vi "StrikerNormal.vi"(6 "atacando ao contrário?":bool=TRUE, 8 "IA Input":T1, 9 "balls":T4[](array[typedef])=[{"x"=-2165.869384765625, "y"=510.4085693359375, "timestamp"=timestamp(2082758857.4639893 s since 1904-01-01), "Vel_x"=0.0, "Vel_y"=0.0}], 10 "Field Size in":T5={"line_width"=10, "field_length"=6000, "field_width"=4000, "boundary_width"=250, "referee_width"=425, "goal_width"=700, "goal_depth"=180, "goal_wall_width"=20, "center_circle_radius"=500, "defense_radius"=500, "defense_stretch"=350, "free_kick_from_defense_dist"=700, "penalty_spot_from_field_line_dist"=450, "penalty_line_from_spot_dist"=350}, 11 "Robot in":T2={"id"=5, "function"=enum."Attacker", "x"=-1842.5054931640625, "y"=520.60986328125, "orientation"=-2.7555055618286133, "v_tangent"=0.0, "v_normal"=0.0, "v_ang"=0.0, "kick_x"=0.0, "kick_z"=0.0, "dribble"=FALSE, "Timestamp"=timestamp(2082758857.4639893 s since 1904-01-01), "dest_x"=0.0, "dest_y"=0.0, "dest_orientation"=0.0, "estimatives"={"est_v_tangent"=0.0, "est_v_normal"=0.0, "est_vx"=0.0, "est_vy"=0.0}}) -> (2 "Robot out":T2={"id"=5, "function"=enum."Attacker", "x"=-1842.5054931640625, "y"=520.60986328125, "orientation"=-2.7555055618286133, "v_tangent"=-0.08361641967936218, "v_normal"=-0.20513016702014014, "v_ang"=0.24456003022714357, "kick_x"=0.0, "kick_z"=0.0, "dribble"=FALSE, "Timestamp"=timestamp(2082758857.4639893 s since 1904-01-01), "dest_x"=0.0, "dest_y"=0.0, "dest_orientation"=0.0, "estimatives"={"est_v_tangent"=0.0, "est_v_normal"=0.0, "est_vx"=0.0, "est_vy"=0.0}})   [LabVIEW 2016]
uses:
  Core/AI Robot.ctl
  Functions Enum.ctl
  Core/Field Size.ctl
  Core/AI Ball.ctl
  Core/AI Input.ctl
  Core/AI Judge.ctl
  Command Enum.ctl
panel:
  in  "dist 2":dbl=700.0
  out "sentido":dbl
  in  "dist":dbl=700.0
  out "Yattacker":dbl
  out "Xattacker":dbl
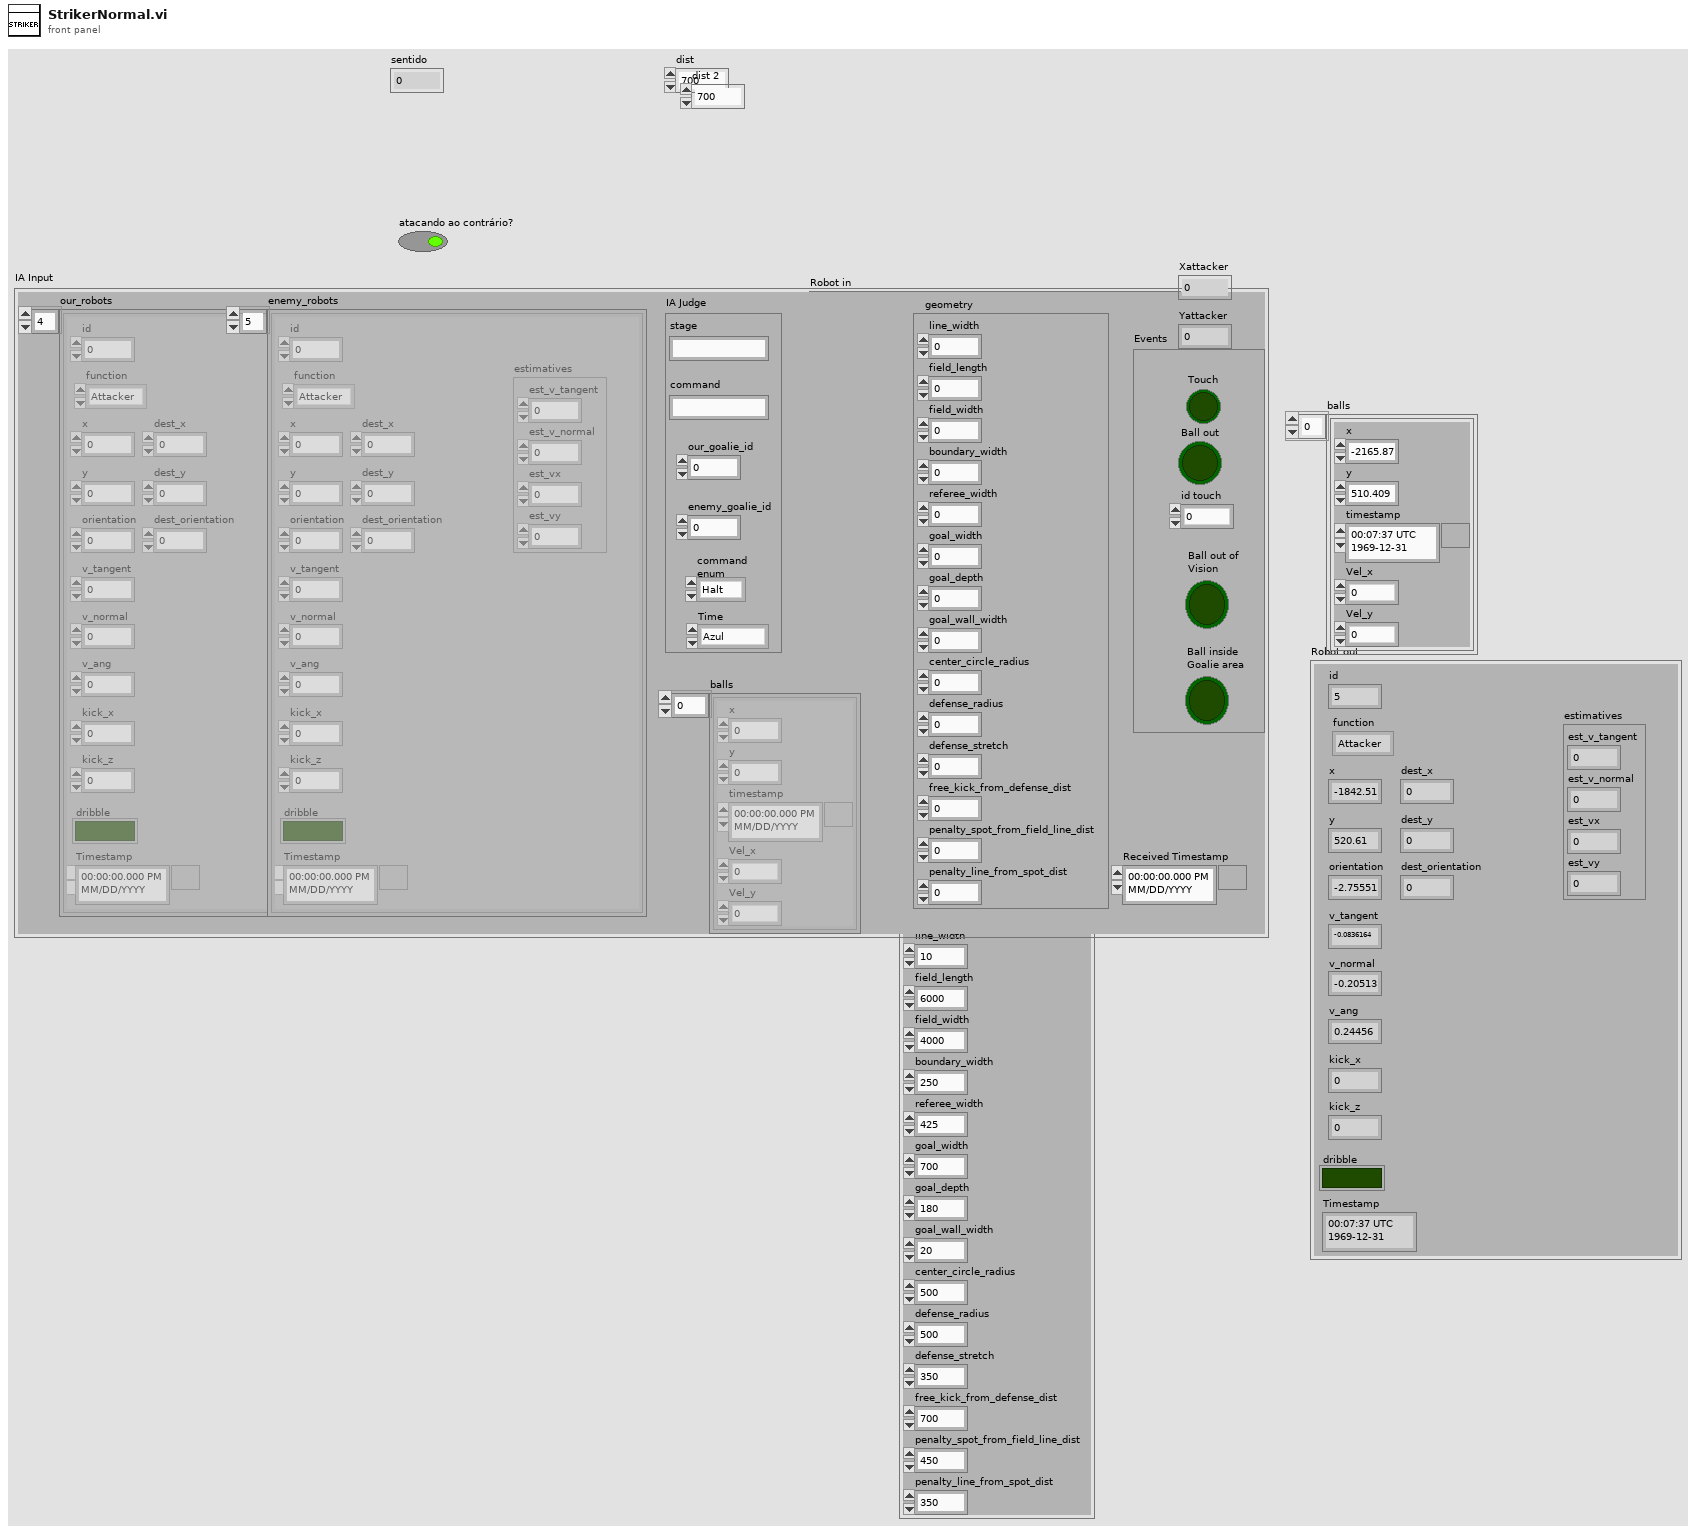
[diagram p1: front panel]
types:
  T1 = typedef "AI Input.ctl" = cluster{"our_robots":T2[], "enemy_robots":T2[], "balls":T4[], "geometry":T5, "IA Judge":T6, "Received Timestamp":timestamp, "Events":cluster{"Touch":bool, "Ball out":bool, "id touch":dbl, "Ball out of \nVision":bool, "Ball inside \nGoalie area":bool}}
  T2 = typedef "AI Robot.ctl" = cluster{"id":u32, "function":T3, "x":dbl, "y":dbl, "orientation":dbl, "v_tangent":dbl, "v_normal":dbl, "v_ang":dbl, "kick_x":dbl, "kick_z":dbl, "dribble":bool, "Timestamp":timestamp, "dest_x":dbl, "dest_y":dbl, "dest_orientation":dbl, "estimatives":cluster{"est_v_tangent":dbl, "est_v_normal":dbl, "est_vx":dbl, "est_vy":dbl}}
  T3 = typedef "Functions Enum.ctl" = enum16{"Attacker", "Goalie", "Defender", "Striker", "Goto 0", "Dummy", "ZigZag"}
  T4 = typedef "AI Ball.ctl" = cluster{"x":dbl, "y":dbl, "timestamp":timestamp, "Vel_x":dbl, "Vel_y":dbl}
  T5 = typedef "Field Size.ctl" = cluster{"line_width":u32, "field_length":u32, "field_width":u32, "boundary_width":u32, "referee_width":u32, "goal_width":u32, "goal_depth":u32, "goal_wall_width":u32, "center_circle_radius":u32, "defense_radius":u32, "defense_stretch":u32, "free_kick_from_defense_dist":u32, "penalty_spot_from_field_line_dist":u32, "penalty_line_from_spot_dist":u32}
  T6 = typedef "AI Judge.ctl" = cluster{"stage":string, "command":string, "our_goalie_id":dbl, "enemy_goalie_id":dbl, "command\nenum":T7, "Time":enum16{"Azul", "Amarelo"}}
  T7 = typedef "Command Enum.ctl" = enum16{"Halt", "Stop", "Force Start", "PKA Normal Start", "Prepare Kickoff Ally", "PKE Normal Start", "Prepare Kickoff Enemy", "Prepare Penalty Ally", "PPA Normal Start", "Prepare Penalty Enemy", "PPE Normal Start", "Direct Free Enemy", "Direct Free Ally", "Indirect Free Enemy", "Indirect Free Ally", "Timeout Enemy", "Timeout Ally", "Goal Enemy", "Goal Ally", "Ball Placement Enemy", "Ball Placement Ally", "None"}
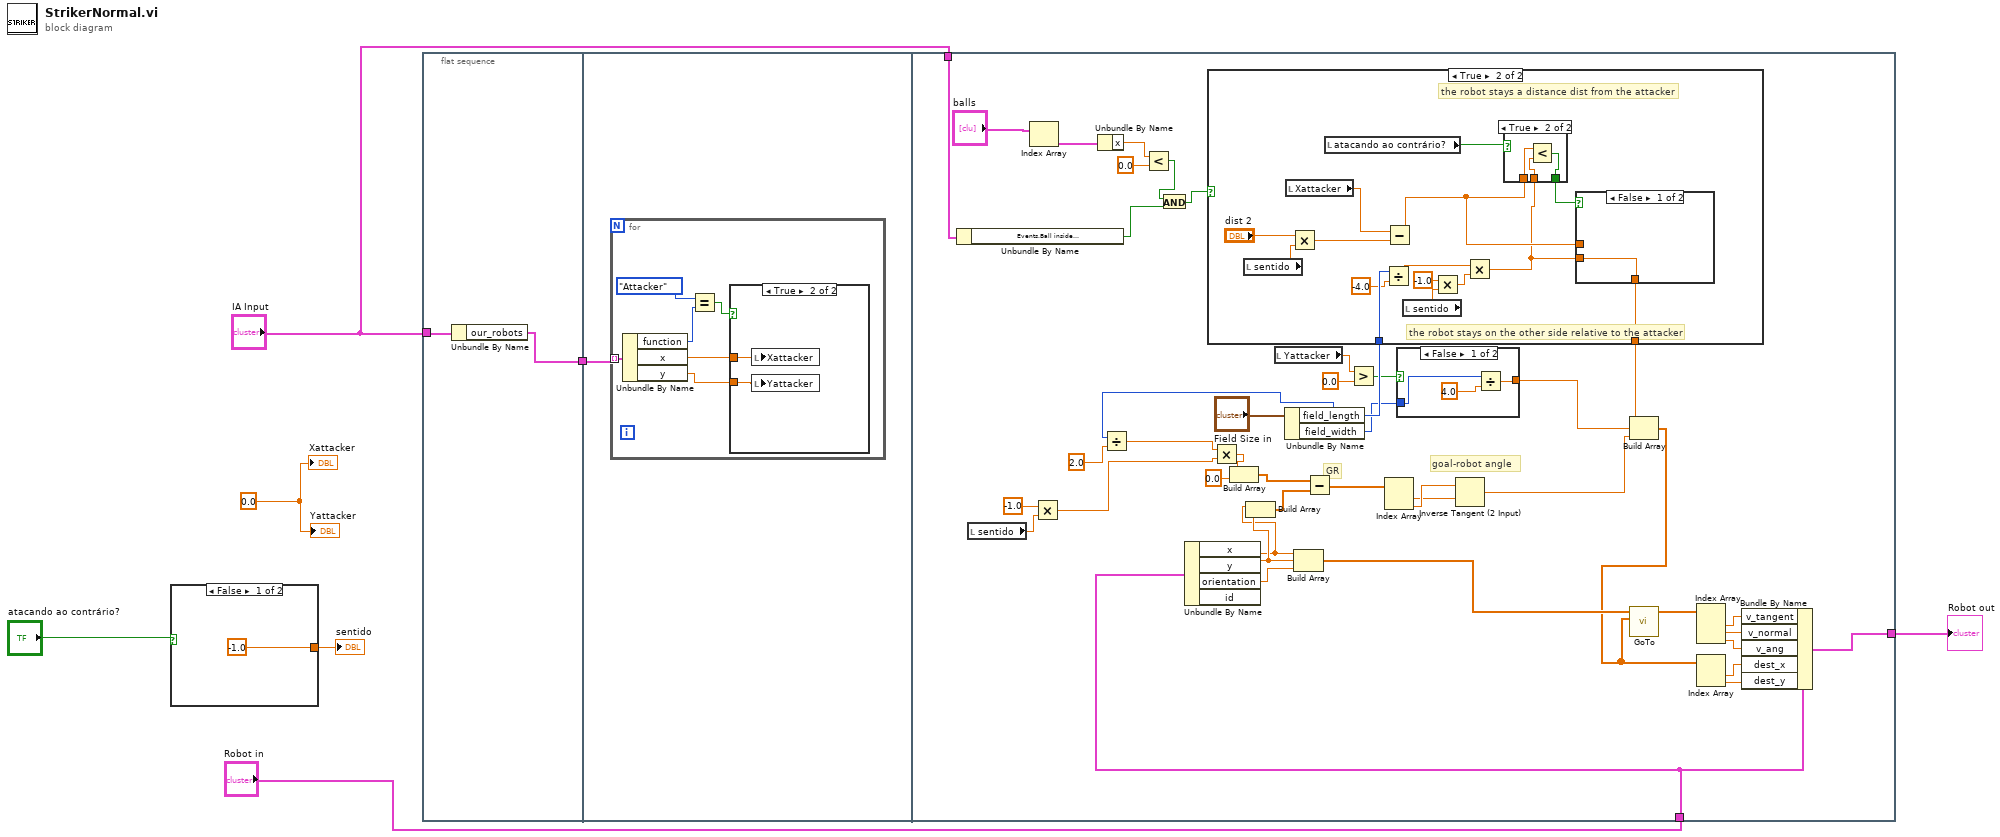
[diagram p0: block diagram]
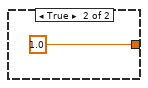
[diagram p2: hidden frame]
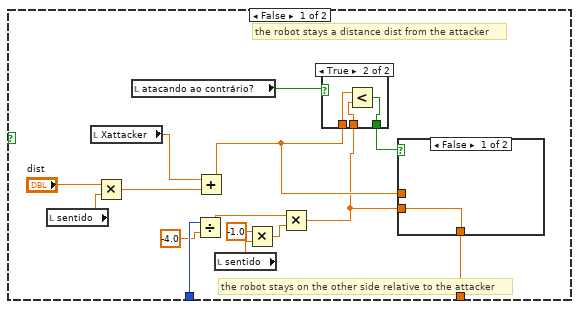
[diagram p4: hidden frame]
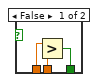
[diagram p5: hidden frame]
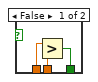
[diagram p7: hidden frame]
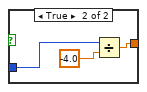
[diagram p9: hidden frame]
diagram:
  w6 = 0.0
  n1 = case shown="False" "atacando ao contrário?" {
    tunnel: [-1.0 1.0] -> w2
    frame False {
    }
    frame True {
    }
  }
  "sentido" <- w2
  n2 = flat-sequence {
    tunnel: "IA Input" -> [w11]
    tunnel: [w10] -> w5
    tunnel: w5 -> [w12]
    tunnel: [w41] -> w7
    tunnel: "Robot in" -> [w39]
    tunnel: "IA Input" -> [w24]
    frame #0 {
      n3 = Unbundle By Name(w11) -> ("our_robots"=w10:T2[])
    }
    frame #1 {
      n4 = for {
        tunnel: w12 -> [w13] mode=indexing
        n5 = Unbundle By Name(w13) -> ("function"=w18:T3, "x"=w15:dbl, "y"=w14:dbl)
        n6 = Equal?(x=Functions_Enum."Attacker", y=w18) -> (x = y?=w16:bool)
        n7 = case shown="True" w16 {
          tunnel: w15 -> [_ w19]
          tunnel: w14 -> [_ w20]
          frame False {
          }
          frame True {
            n8 = local write "Xattacker"(w19) -> ()
            n9 = local write "Yattacker"(w20) -> ()
          }
        }
      }
    }
    frame #2 {
      # "GR"
      # "goal-robot angle"
      n10 = Unbundle By Name(w24) -> ("Events.Ball inside \nGoalie area"=w21:bool)
      n11 = local read "sentido"() -> (w37:dbl)
      n12 = Index Array(array="balls") -> (element=w27:T4)  [unwired: 1 in]
      n13 = Multiply(x=-1.0, y=w37) -> (x*y=w36:dbl)
      n14 = Unbundle By Name(w27) -> ("x"=w26:dbl)
      n15 = Less?(x=w26, y=0.0) -> (x < y?=w22:bool)
      n16 = And(x=w22, y=w21) -> (x .and. y?=w23:bool)
      n17 = Unbundle By Name(w39) -> ("x"=w55:dbl, "y"=w56:dbl, "orientation"=w42:dbl)  [unwired: 1 out]
      n18 = Build Array(w55, w56) -> (w57:dbl[])
      n19 = local read "Yattacker"() -> (w40:dbl)
      n20 = Unbundle By Name("Field Size in") -> ("field_length"=w59:u32, "field_width"=w46:u32)
      n21 = Divide(x=w59, y=2.0) -> (x/y=w35:dbl)
      n22 = case shown="True" w23 {
        tunnel: w59 -> [w77 w100]
        tunnel: [w76 w99] -> w48
        frame False {
          # "the robot stays on the other side relative to the attacker"
          # "the robot stays a distance dist from the attacker"
          n23 = local read "sentido"() -> (w67:dbl)
          n24 = local read "Xattacker"() -> (w73:dbl)
          n25 = Multiply(x="dist", y=w67) -> (x*y=w72:dbl)
          n26 = local read "atacando ao contrário?"() -> (w66:bool)
          n27 = Divide(x=w77, y=-4.0) -> (x/y=w74:dbl)
          n28 = Add(x=w73, y=w72) -> (x+y=w65:dbl)
          n29 = local read "sentido"() -> (w70:dbl)
          n30 = Multiply(x=-1.0, y=w70) -> (x*y=w69:dbl)
          n31 = Multiply(x=w74, y=w69) -> (x*y=w64:dbl)
          n32 = case shown="True" w66 {
            tunnel: w65 -> [w80 w82]
            tunnel: w64 -> [w79 w83]
            tunnel: [w78 w81] -> w63
            frame False {
              n33 = Greater?(x=w80, y=w79) -> (0:w78:bool)
            }
            frame True {
              n34 = Less?(x=w82, y=w83) -> (x < y?=w81:bool)
            }
          }
          n35 = case shown="False" w63 {
            tunnel: [w84 w85] -> w76
            tunnel: w65 -> [_ w85]
            tunnel: w64 -> [w84 _]
            frame False {
            }
            frame True {
            }
          }
        }
        frame True {
          # "the robot stays on the other side relative to the attacker"
          # "the robot stays a distance dist from the attacker"
          n36 = local read "sentido"() -> (w90:dbl)
          n37 = local read "Xattacker"() -> (w96:dbl)
          n38 = Multiply(x="dist 2", y=w90) -> (x*y=w95:dbl)
          n39 = local read "atacando ao contrário?"() -> (w89:bool)
          n40 = Divide(x=w100, y=-4.0) -> (x/y=w97:dbl)
          n41 = Subtract(x=w96, y=w95) -> (x-y=w88:dbl)
          n42 = local read "sentido"() -> (w93:dbl)
          n43 = Multiply(x=-1.0, y=w93) -> (x*y=w92:dbl)
          n44 = Multiply(x=w97, y=w92) -> (x*y=w87:dbl)
          n45 = case shown="True" w89 {
            tunnel: w88 -> [w103 w105]
            tunnel: w87 -> [w102 w106]
            tunnel: [w101 w104] -> w86
            frame False {
              n46 = Greater?(x=w103, y=w102) -> (0:w101:bool)
            }
            frame True {
              n47 = Less?(x=w105, y=w106) -> (x < y?=w104:bool)
            }
          }
          n48 = case shown="False" w86 {
            tunnel: [w107 w108] -> w99
            tunnel: w88 -> [_ w108]
            tunnel: w87 -> [w107 _]
            frame False {
            }
            frame True {
            }
          }
        }
      }
      n49 = Multiply(x=w35, y=w36) -> (x*y=w34:dbl)
      n50 = Build Array(w34, 0.0 ("element")) -> (w61:dbl[])
      n51 = Build Array(w55, w56, w42) -> (w32:dbl[])
      n52 = Subtract(x=w61, y=w57) -> (x-y=w54:dbl[])
      n53 = Greater?(x=w40, y=0.0) -> (0:w43:bool)
      n54 = Index Array(array=w54) -> (element #1=w52:dbl, element #2=w53:dbl)  [unwired: 2 in]
      n55 = case shown="False" w43 {
        tunnel: [w110 w113] -> w47
        tunnel: w46 -> [w109 w112]
        frame False {
          n56 = Divide(x=w109, y=4.0) -> (x/y=w110:dbl)
        }
        frame True {
          n57 = Divide(x=w112, y=-4.0) -> (x/y=w113:dbl)
        }
      }
      n58 = Inverse Tangent (2 Input)(1:w52, 2:w53) -> (0:w62:dbl)
      n59 = Build Array(w48, w47, w62) -> (w29:dbl[])
      n60 = call "GoTo.vi"("Target"=w29, "Position"=w32) -> ("Output\nVelocity"=w33:dbl[])  [unwired: 8 in, 1 out]
      n61 = Index Array(array=w33) -> (element #1=w49:dbl, element #2=w51:dbl, element #3=w50:dbl)  [unwired: 3 in]
      n62 = Index Array(array=w29) -> (element #1=w31:dbl, element #2=w30:dbl)  [unwired: 2 in]
      n63 = Bundle By Name(cluster=w39, "v_tangent"=w49, "v_normal"=w51, "v_ang"=w50, "dest_x"=w31, "dest_y"=w30) -> (w41:T2)
    }
  }
  "Robot out" <- w7
  "Xattacker" <- w6
  "Yattacker" <- w6
